vi "SeCrTs-RD AI config Divider.vi"(11 "AI config":T1(array[cluster])) -> (2 "AI V":T1(array[cluster]), 3 "AI C":T1(array[cluster]))   [LabVIEW 2022 SP3]
panel:
  in  "V_DAQ Card":string="PXI1Slot9"
  in  "C_DAQ Card":string="PXI1Slot3"
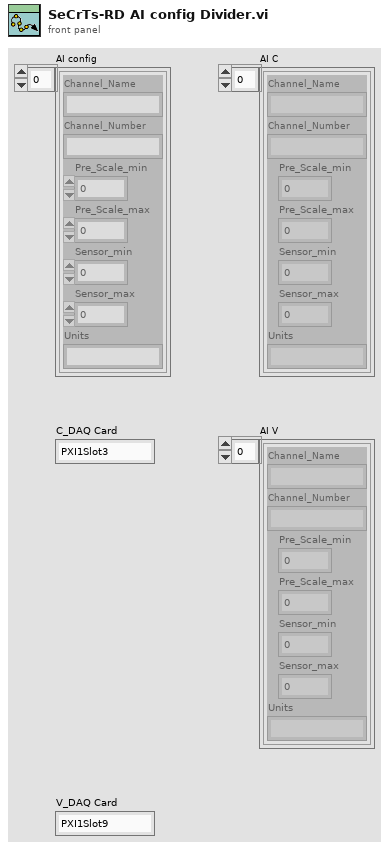
[diagram p1: front panel]
types:
  T1 = cluster{"Channel_Name":string, "Channel_Number":string, "Pre_Scale_min":dbl, "Pre_Scale_max":dbl, "Sensor_min":dbl, "Sensor_max":dbl, "Units":string}[]
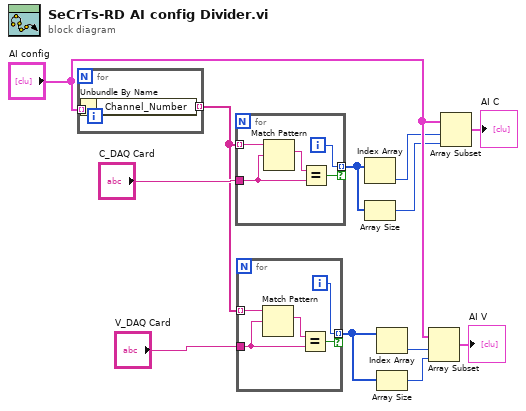
[diagram p0: block diagram]
diagram:
  n1 = for {
    tunnel: "AI config" -> [w14] mode=indexing
    tunnel: [w13] -> w8 mode=indexing
    n2 = Unbundle By Name(w14) -> ("Channel_Number"=w13:string)
  }
  n3 = for {
    tunnel: w8 -> [w15] mode=indexing
    tunnel: "C_DAQ Card" -> [w18]
    tunnel: [w17] -> w2 mode=indexing if=w16
    i -> [w17]
    n4 = Match Pattern(string=w15, regular expression=w18) -> (match substring=w19:string)  [unwired: 1 in, 3 out]
    n5 = Equal?(x=w19, y=w18) -> (x = y?=w16:bool)
  }
  n6 = for {
    tunnel: "V_DAQ Card" -> [w20]
    tunnel: w8 -> [w23] mode=indexing
    tunnel: [w22] -> w5 mode=indexing if=w21
    i -> [w22]
    n7 = Match Pattern(string=w23, regular expression=w20) -> (match substring=w24:string)  [unwired: 1 in, 3 out]
    n8 = Equal?(x=w24, y=w20) -> (x = y?=w21:bool)
  }
  n9 = Index Array(array=w2) -> (element=w3:i32)  [unwired: 1 in]
  n10 = Array Size(array=w2) -> (size(s)=w1:i32)
  n11 = Index Array(array=w5) -> (element=w6:i32)  [unwired: 1 in]
  n12 = Array Size(array=w5) -> (size(s)=w7:i32)
  n13 = Array Subset(array="AI config", index=w6, length=w7) -> (→"AI V":T1)
  n14 = Array Subset(array="AI config", index=w3, length=w1) -> (→"AI C":T1)
